vi "Get Pixel Intensity Array_Luan2024.05.01.vi"(3 "error in (no error)":errorcluster, 4 "Selected line":i32=300, 5 "Image":T2(plugin-control)) -> (0 "error out":errorcluster, 1 "Intensity vs Pixel":u8[](graph), 2 "ROI Descriptor":T1 {"Contours"."Type" items=["No Selection", "Point", "Line", "Rectangle", "Oval", "Polygon", "Freehand Region", "Annulus", "Unused2", "Unused3", "Broken Line", "Freehand Line", "Rotated Rectangle"]})   [LabVIEW 2023]
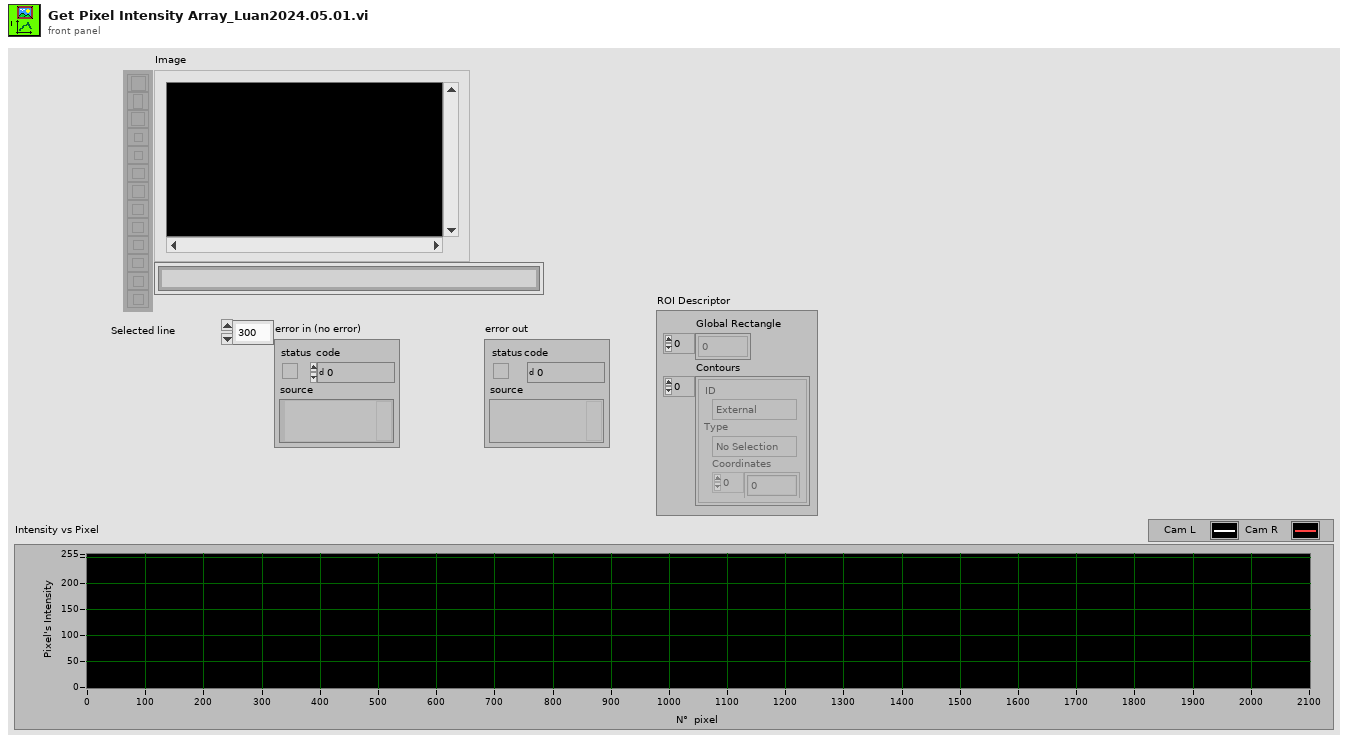
[diagram p1: front panel]
types:
  T1 = typedef "ROI Descriptor" = cluster{"Global Rectangle":i32[], "Contours":cluster{"ID":enum32{"External", "Internal"}, "Type":u32, "Coordinates":i32[]}[]}
  T2 = typedef "IMAQ Image.ctl" = refnum<image>
  T3 = typedef "IMAQ Line" = cluster{"Start X":i32, "Start Y":i32, "End X":i32, "End Y":i32}
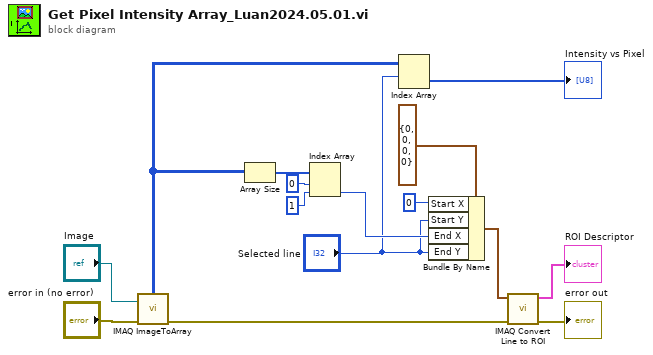
[diagram p0: block diagram]
diagram:
  n1 = call "IMAQ ImageToArray"("error in (no error)"="error in (no error)", "Image"="Image") -> ("error out"=w3:errorcluster, "Image Pixels (U8)"=w7:u8[][])  [unwired: 2 in, 3 out]
  n2 = Array Size(array=w7) -> (size(s)=w12:i32[])
  n3 = Index Array(array=w12, index #1=0 ("index"), index #2=1 ("index")) -> (element #2=w11:i32)  [unwired: 1 out]
  n4 = Index Array(array=w7, index (row)="Selected line") -> (element=→"Intensity vs Pixel":u8[])  [unwired: 1 in]
  n5 = Bundle By Name(cluster=T3 {"Start X"=0, "Start Y"=0, "End X"=0, "End Y"=0} ("Line"), "Start X"=0, "Start Y"="Selected line", "End X"=w11, "End Y"="Selected line") -> (w1:T3)
  n6 = call "IMAQ Convert Line to ROI"("error in (no error)"=w3, "Line"=w1) -> ("error out"=→"error out":errorcluster, "ROI Descriptor"=→"ROI Descriptor":T1)  [unwired: 7 in]
